vi "PD_Controller.vi"(8 "PD Gain":cluster{"Kd":dbl, "Kp":dbl}={"Kd"=0.1894, "Kp"=0.0}, 9 "dt":dbl, 10 "Error (n-1)":dbl, 11 "Error":dbl) -> (2 "V":dbl, 3 "Error Out":dbl)   [LabVIEW 2022 SP3]
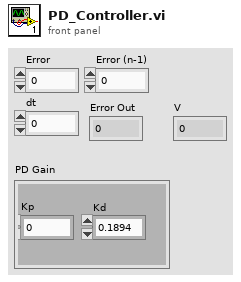
[diagram p1: front panel]
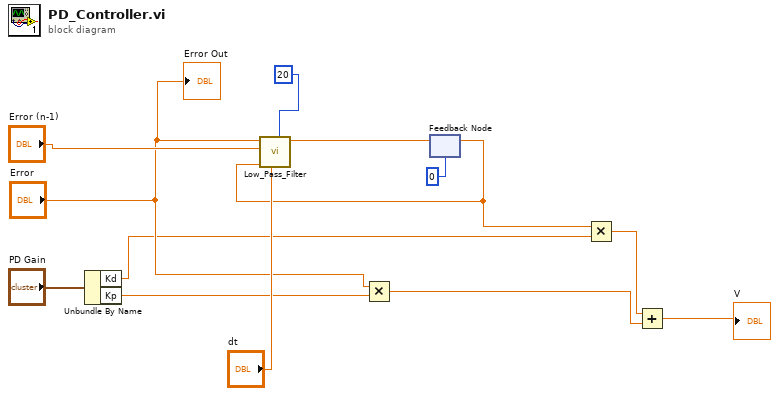
[diagram p0: block diagram]
diagram:
  n1 = Unbundle By Name("PD Gain") -> ("Kd"=w4:dbl, "Kp"=w7:dbl)
  n2 = Multiply(x="Error", y=w7) -> (x*y=w2:dbl)
  n3 = feedback #1(0) -> (w5:dbl)
  n4 = call "Low_Pass_Filter.vi"("Cut-Off Frequency"=20, "Sampling Interval"="dt", "Previous Output"=w5, "Previous Input"="Error (n-1)", "Current Input"="Error") -> ("Derivative"=w10:dbl)  [unwired: 6 in]
  n5 = feedback-in #1(w10) -> ()
  n6 = Multiply(x=w5, y=w4) -> (x*y=w3:dbl)
  n7 = Add(x=w3, y=w2) -> (x+y=→"V":dbl)
  "Error Out" <- "Error"
